vi "Z Aux Read U File.vi"(8 "error in (no error)":errorcluster caption="错误输入（无错误）", 9 "pinum":i32, 10 "pVarlist":sgl[](array[numeric])=array[4097 elements], 11 "sFilename":string) -> (0 "error out":errorcluster caption="错误输出", 1 "pinum out":i32, 2 "pVarlist out":sgl[](array[numeric]), 3 "function return":i32)   [LabVIEW 2015, in "zauxdll.lvlib"]
doc: "int32 __stdcall ZAux_ReadUFile(const char *sFilename, float pVarlist[], int* pinum);"
uses:
  zauxdll.lvlib
  Radar - 2015 32bit_autoqueue_angle_0319/zauxdll-2014/zauxdll.dll
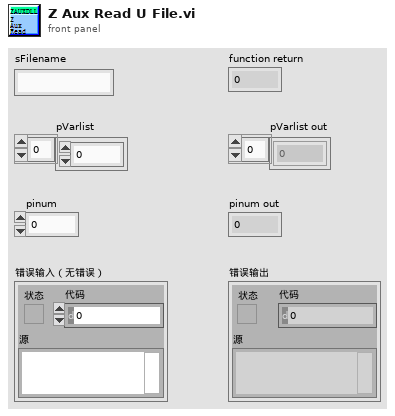
[diagram p1: front panel]
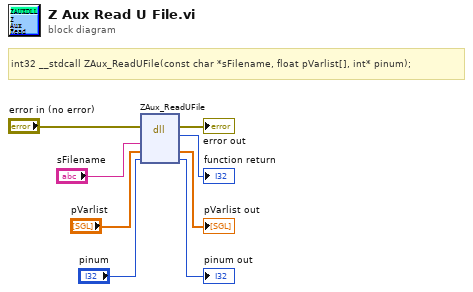
[diagram p0: block diagram]
diagram:
  # "int32 __stdcall ZAux_ReadUFile(const char *sFilename, float pVarlist[], int* pinum);"
  n1 = dll-call lib="D:/vicomm case/cub/0717/Radar - 2015 32bit_autoqueue_angle_0319/zauxdll-2014/zauxdll.*" fn="ZAux_ReadUFile"(error in="error in (no error)", "sFilename"="sFilename", "pVarlist"="pVarlist", "pinum"="pinum") -> (error out=→"error out":errorcluster, →"function return":i32, "pVarlist"=→"pVarlist out":sgl[], "pinum"=→"pinum out":i32)  [unwired: 3 in, 1 out]
